vi "reprGraphical.vi"(8 "error in (no error)":errorcluster, 9 "Image Descriptor":T1={"Upper-Left Corner Coordinates"={"UTM Zone"=0.0, "Hemisphere"=enum."North", "East"=0.0, "North"=0.0}, "Meters/Pixel"=42.294203} {"Upper-Left Corner Coordinates"."North" format="%#_10f"; "Upper-Left Corner Coordinates"."East" format="%#_8f"}, 10 "Image In":T3, 11 "Idle in":refnum<class "Idle.lvclass">) -> (0 "error out":errorcluster, 2 "Image Out":T3, 3 "Idle out":refnum<class "Idle.lvclass">)   [LabVIEW 2011, in "Idle.lvclass"]
uses:
  Idle.lvclass
  <vilib>/vision/Image Controls.llb/IMAQ Image.ctl
  0-OCU/0 Code/mission input/0-Image Descriptor.ctl
  2 Typedefs/UTM Location.ctl
  Idle.lvclass/Idle.ctl
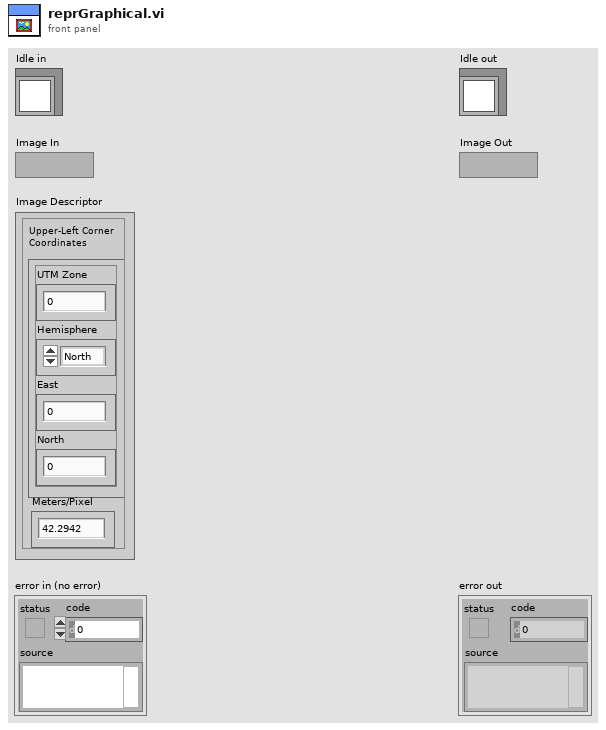
[diagram p1: front panel]
types:
  T1 = typedef "0-Image Descriptor.ctl" = cluster{"Upper-Left Corner Coordinates":T2, "Meters/Pixel":dbl}
  T2 = typedef "UTM Location.ctl" = cluster{"UTM Zone":dbl, "Hemisphere":enum16{"North", "South"}, "East":dbl, "North":dbl}
  T3 = typedef "IMAQ Image.ctl" = refnum<image>
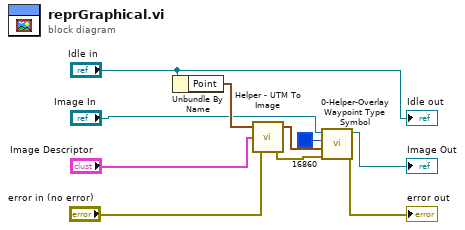
[diagram p0: block diagram]
diagram:
  n1 = Unbundle By Name("Idle in") -> ("Point"=w10:T2)
  n2 = call "Helper - UTM To Image.vi"("error in"="error in (no error)", "Image Descriptor"="Image Descriptor", "UTM Location"=w10) -> ("error out"=w1:errorcluster, "Pixel Coordinates"=w7:cluster{"X":i32, "Y":i32})  [unwired: 1 out]
  n3 = call "0-Helper-Overlay Waypoint Type Symbol.vi"("error in"=w1, "Overlay Location"=w7, "Icon Color"=u32 16860, "Image in"="Image In") -> ("error out"=→"error out":errorcluster, "Image out"=→"Image Out":T3)  [unwired: 6 in]
  "Idle out" <- "Idle in"
